vi "Pause.vi"(8 "error in (no error)":errorcluster, 11 "ASIA Pump C Settings in":T1) -> (0 "error out":errorcluster, 2 "Task Completed":bool=TRUE, 3 "ASIA Pump C Settings out":T1)   [LabVIEW 2018, in "ASIA Pump.lvlib"]
uses:
  ASIA Pump.lvlib
  Pump Settings.ctl
panel:
  out "path out":path
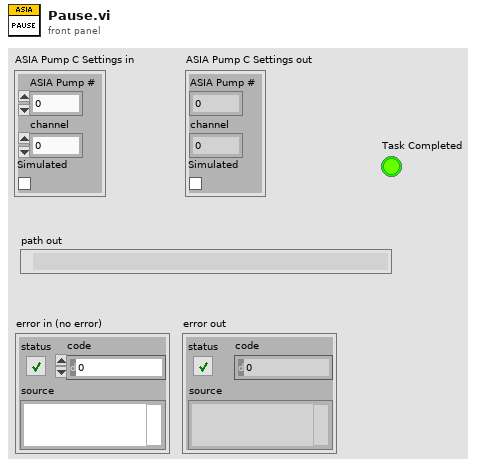
[diagram p1: front panel]
types:
  T1 = typedef "ASIA Pump.lvlib/Pump Settings.ctl" = cluster{"ASIA Pump #":i32, "channel":i32, "Simulated":bool}
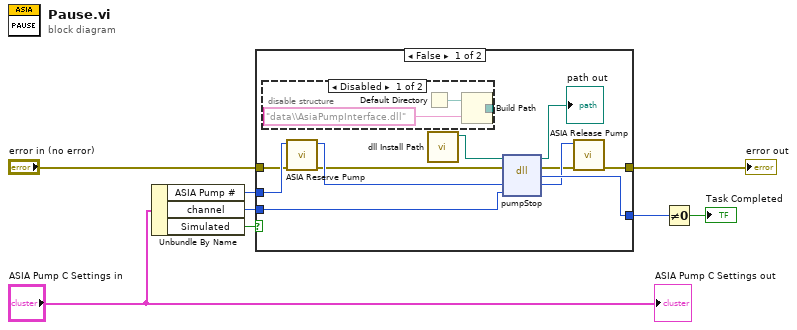
[diagram p0: block diagram]
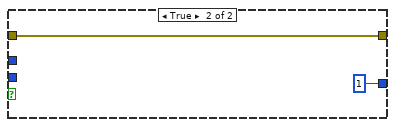
[diagram p3: hidden frame]
diagram:
  n1 = Unbundle By Name("ASIA Pump C Settings in") -> ("ASIA Pump #"=w3:i32, "channel"=w2:i32, "Simulated"=w1:bool)
  n2 = case shown="False" w1 {
    tunnel: w3 -> [w16 _]
    tunnel: w2 -> [w19 _]
    tunnel: "error in (no error)" -> [w14 w24]
    tunnel: [w12 w24] -> w6
    tunnel: [w18 u8 1 ("Bool")] -> w5
    frame False {
      n3 = disable-structure shown="Disabled" {
        disable-tunnel: [w20 _] -> _
        frame Disabled {
          n4 = Default Directory() -> (w21:path)
          n5 = Build Path(base path=w21, name or relative path="data\\AsiaPumpInterface.dll") -> (appended path=w20:path)
        }
        frame Enabled {
        }
      }
      n6 = call "ASIA Reserve Pump.vi"("error in (no error)"=w14, "ASIA Pump # In"=w16) -> ("error out"=w15:errorcluster, "ASIA Pump # Out"=w17:i32)  [unwired: 8 in]
      n7 = call "dll Install Path.vi"() -> ("system directory"=w10:path)  [unwired: 11 in]
      n8 = dll-call lib="C:/Program Files (x86)/Pfizer/FAST/data/AsiaPumpInterface.dll" fn="pumpStop"(path in=w10, error in=w15, "pumpNum"=w17, "channel"=w19) -> (path out=→"path out":path, error out=w11:errorcluster, "Bool"=w18:u8, "pumpNum"=w13:u32)  [unwired: 2 in]
      n9 = call "ASIA Release Pump.vi"("error in (no error)"=w11, "pumpNum"=w13) -> ("error out"=w12:errorcluster)  [unwired: 8 in, 1 out]
    }
    frame True {
    }
  }
  "error out" <- w6
  n10 = Not Equal To 0?(x=w5) -> (x != 0?=→"Task Completed":bool)
  "ASIA Pump C Settings out" <- "ASIA Pump C Settings in"
